vi "Motor Off.vi"(8 "error in (no error)":errorcluster, 11 "VISA resource name":refnum<visa-resource-name>) -> (0 "error out":errorcluster, 3 "VISA resource name out":refnum<visa-resource-name>)   [LabVIEW 2024, in "Revidyne Generator.lvlib"]
doc: "This VI will cause the generator to start moving."
uses:
  Revidyne Generator.lvlib
  45d63ee6-6c00-45e0-ac99-6ec58d3744cf.vi
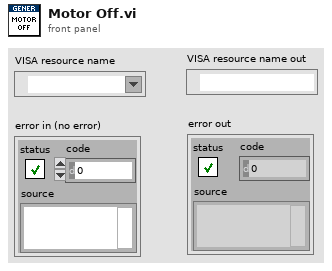
[diagram p1: front panel]
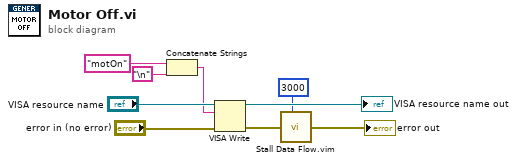
[diagram p0: block diagram]
diagram:
  n1 = Concatenate Strings("motOn" ("command"), "\n") -> (w6:string)
  n2 = VISA Write(VISA resource name="VISA resource name", write buffer=w6, error in (no error)="error in (no error)") -> (VISA resource name out=→"VISA resource name out":refnum<visa-resource-name>, error out=w3:errorcluster)  [unwired: 1 out]
  n3 = call "Stall Data Flow.vim"("value in"=w3, "milliseconds to wait"=u32 3000) -> ("value out"=→"error out":errorcluster)  [unwired: 1 out]
